vi "XIPIN_AXI_Interconnect_RTL_1_7.vi"   [LabVIEW 2017]
doc: "The AXI Interconnect core connects one or more AXI4 memory-mapped master devices to one AXI4 slave device.\n------------------------------------\n<b>Need License</b> : No\n<b>Interface</b> : AXI4"
uses:
  <vilib>/rvi/XilinxIP/XIPIN_XNode/niFpgaXIPIN.xnode
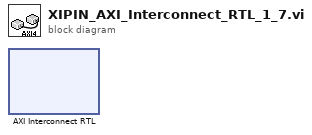
[diagram p0: block diagram]
diagram:
  n1 = xnode ("AXI Interconnect RTL")() -> ()
